vi "Reset Files.vi"(8 "error in":errorcluster, 11 "Peer Review in":refnum<class "Peer Review.lvclass">) -> (0 "error out":errorcluster, 3 "Peer Review out":refnum<class "Peer Review.lvclass">)   [LabVIEW 2020, in "Peer Review.lvclass"]
uses:
  Peer Review.lvclass
  Peer Review.lvclass/Peer Review.ctl
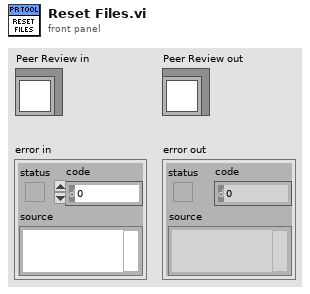
[diagram p1: front panel]
types:
  T1 = typedef "Peer Review.lvclass/File Info.ctl" = cluster{"File ID":i32, "Commit ID":i32, "Reviewed Hash":string, "Relative Path":string, "File Path":path, "File Checksum":string, "State":T2, "FP Changes":i32, "BD Changes":i32, "FP Bounds Error":dbl, "BD Bounds Error":dbl, "Lines Added":i32, "Lines Removed":i32, "Analysis Passes":i32, "Analysis Fails":i32, "Attribute Changes":i32, "Reentrancy Changes":string, "Cyclomatic Complexity":i32, "Node Count":u32, "Revision Number":u32, "LabVIEW Version":string, "Description":string, "Master Path":path, "Master Checksum":string, "VI Type":T3, "LabVIEW File":bool, "Review Complete":bool, "File Ref":refnum<vi>}
  T2 = typedef "Peer Review.lvclass/File State.ctl" = enum16{"Interrogation Needed", "Modified", "Deleted", "Added", "Matches Previous", "No Changes", "Moved"}
  T3 = typedef "Peer Review.lvclass/VI Type.ctl" = enum32{"invalid VI type", "Standard VI", "Control VI", "Global VI", "Polymorphic VI", "Configuration VI", "SubSystem", "Facade VI", "Method VI", "Statechart Diagram VI"}
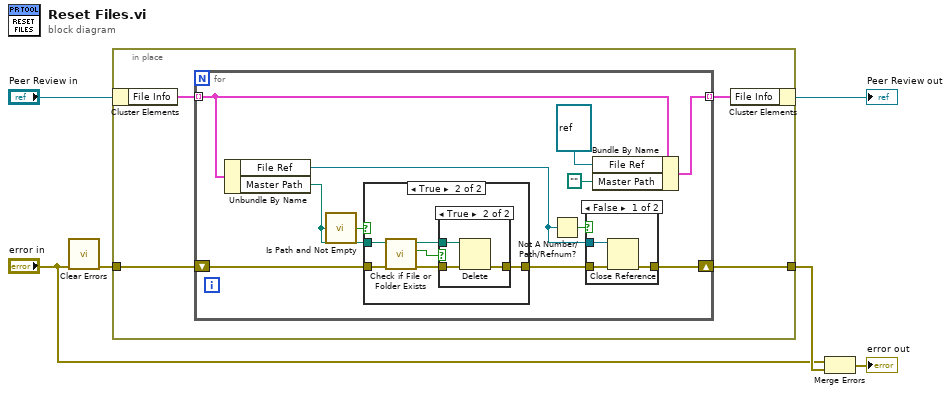
[diagram p0: block diagram]
diagram:
  n1 = call <vilib>:"Clear Errors.vi"("error in (no error)"="error in") -> ("error out"=w4:errorcluster)  [unwired: 5 in, 1 out]
  n2 = in-place {
    in-place-border: w4 -> [w7]
    in-place-border: [w8] -> w3
    n3 = in-place-cluster #1("Peer Review in") -> ("File Info"=w10:T1[])
    n4 = for {
      tunnel: w10 -> [w16] mode=indexing
      tunnel: [w13] -> w9 mode=indexing
      shift-right: [w11] -> w8
      shift-left: w7 -> [w21]
      n5 = Unbundle By Name(w16) -> ("File Ref"=w17:refnum<vi>, "Master Path"=w20:path)
      n6 = call <vilib>:"Is Path and Not Empty.vi"("path"=w20) -> ("Is Path and Not Empty?"=w19:bool)  [unwired: 4 in]
      n7 = case shown="True" w19 {
        tunnel: w21 -> [w22 w27]
        tunnel: w20 -> [_ w25]
        tunnel: [w22 w24] -> w12
        frame False {
        }
        frame True {
          n8 = call <vilib>:"Check if File or Folder Exists.vi"("error in (no error)"=w27, "path"=w25) -> ("error out"=w26:errorcluster, "file or folder exists?"=w23:bool, "dup path"=w28:path)  [unwired: 7 in]
          n9 = case shown="True" w23 {
            tunnel: w28 -> [_ w32]
            tunnel: w26 -> [w29 w31]
            tunnel: [w29 w30] -> w24
            frame False {
            }
            frame True {
              n10 = Delete(path (use dialog)=w32, error in=w31) -> (error out=w30:errorcluster)  [unwired: 3 in, 2 out]
            }
          }
        }
      }
      n11 = Not A Number/Path/Refnum?(number/path/refnum=w17) -> (NaN/Path/Refnum?=w18:bool)
      n12 = case shown="False" w18 {
        tunnel: w17 -> [w35 _]
        tunnel: [w34 w36] -> w11
        tunnel: w12 -> [w33 w36]
        frame False {
          n13 = Close Reference(reference=w35, error in (no error)=w33) -> (error out=w34:errorcluster)
        }
        frame True {
        }
      }
      n14 = Bundle By Name(cluster=w16, "File Ref"=refnum<vi> refnum, "Master Path"=path "") -> (w13:T1)
    }
    n15 = in-place-cluster #1("File Info"=w9) -> (→"Peer Review out":refnum<class "Peer Review.lvclass">)
  }
  n16 = Merge Errors("error in", w3) -> (→"error out":errorcluster)
